vi "NumArray to CatStr.vi"(1 "Array":i8[](array[numeric])) -> (0 "spreadsheet string":string)   [LabVIEW 2019]
panel:
  out "number of replacements":i32
  out "result string":string
  out "spreadsheet string 2":string
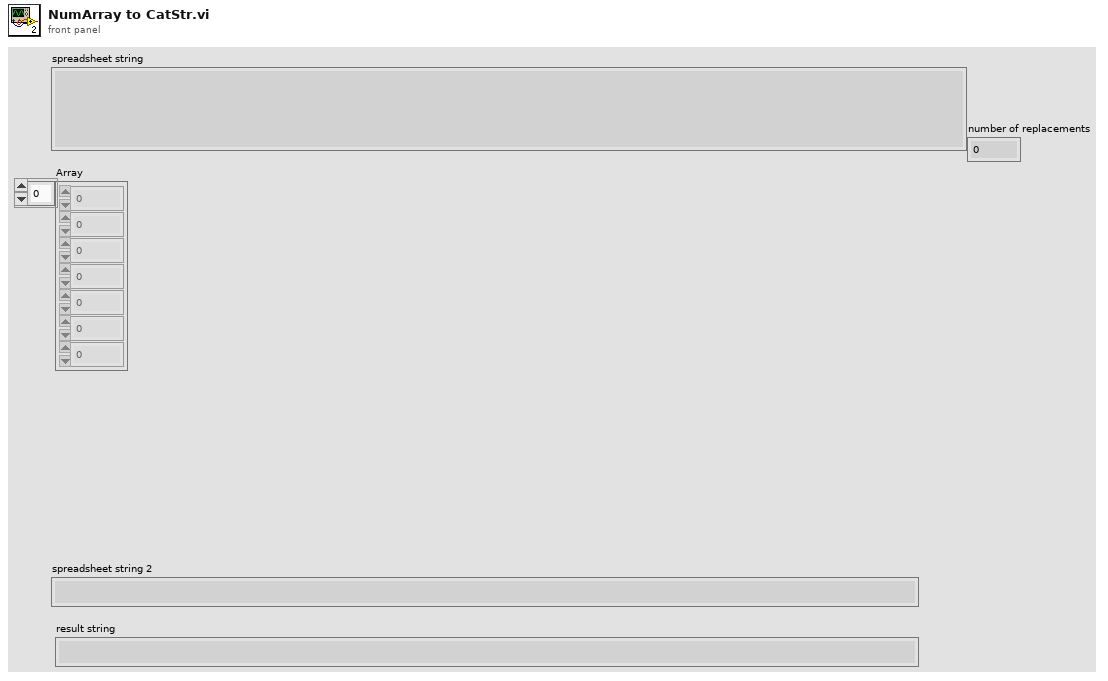
[diagram p1: front panel]
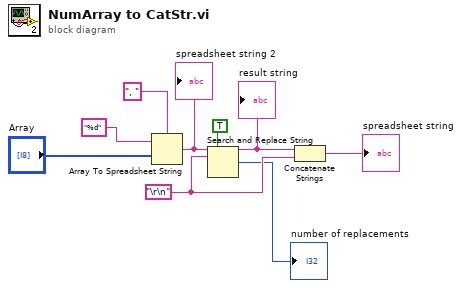
[diagram p0: block diagram]
diagram:
  w3 = "\r\n"
  n1 = Array To Spreadsheet String(delimiter (Tab)=", ", array="Array", 3:"%d" ("format string")) -> (spreadsheet string=w6:string)
  "spreadsheet string 2" <- w6
  n2 = Search and Replace String(replace all?=TRUE ("replace all? (F)"), input string=w6, search string=w3) -> (result string=w5:string, number of replacements=→"number of replacements":i32)  [unwired: 5 in, 2 out]
  "result string" <- w5
  n3 = Concatenate Strings(w5, w3) -> (→"spreadsheet string":string)
